vi "blank cursor.vi"   [LabVIEW 2010]
uses:
  <vilib>/Utility/cursorutil.llb/Set Cursor (Cursor ID).vi
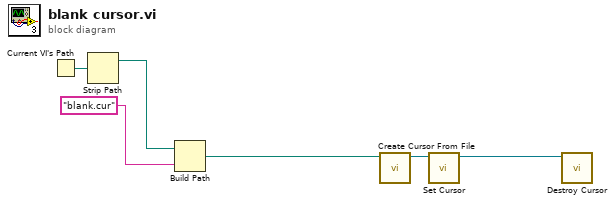
[diagram p0: block diagram]
diagram:
  n1 = Current VI's Path() -> (path=w6:path)
  n2 = Strip Path(path=w6) -> (stripped path=w5:path)  [unwired: 1 out]
  n3 = Build Path(base path=w5, name or relative path="blank.cur") -> (appended path=w3:path)
  n4 = call <vilib>:"Create Cursor From File.vi"("cursor file"=w3) -> ("cursor ID"=w2:refnum<k1>)  [unwired: 9 in, 1 out]
  n5 = call-poly <vilib>:"Set Cursor.vi"("cursor ID"=w2) -> ("previous cursor ID"=w1:refnum<k1>)  [unwired: 9 in, 1 out]
  n6 = call <vilib>:"Destroy Cursor.vi"("cursor ID"=w1) -> ()  [unwired: 9 in, 1 out]
